vi "SistemaCalentadorAgua.vi"() -> ()   [LabVIEW 2010]
uses:
  <vilib>/Platform/TimedLoop/XDataNode/XDataNode.xnode
  <vilib>/Platform/TimedLoop/XDataNode/timing_clust.ctl
  <vilib>/Platform/TimedLoop/XDataNode/nitl_modes.ctl
  <vilib>/Platform/TimedLoop/XDataNode/wakeup.ctl
  <vilib>/Instr/_visa.llb/VISA Configure Serial Port (Instr).vi
  <vilib>/Platform/TimedLoop/XDataNode/XDNodeRunTimeDep.lvlib
panel:
  out "Waveform Chart 2":i16(graph)
  in  "Ajuste":i16(slide) scale=0.0..10.0
  out "Waveform Chart":dynamicdata(graph)
  out "Temp Actual":i16(slide) scale=20.0..60.0
  in  "Set- Point\n       Temperatura 2":i16(slide) scale=20.0..60.0
  out "off":bool
  out "on":bool
  in  "Manual/Automatico":bool
  in  "Set- Point Potencia (W)":i16(slide) scale=0.0..400.0
  out "valvula":bool
  out "Caldera":dbl(slide) scale=0.0..10.0
  in  "Period                :":i64=1000
  in  "Flow control    :":u16(ring) items=["None"=0, "XON/XOFF"=1, "RTS/CTS"=2, "DTR/DSR"=4]
  in  "Stop bits         :":u16(ring)=10 items=["1.0"=10, "1.5"=15, "2.0"=20]
  in  "Paridad            :":u16(ring) items=["None", "Odd", "Even", "Mark", "Space"]
  in  "Data bits          :":u16=8 min=5 max=8 step=1
  in  "VISA resource : name:":refnum<visa-resource-name>="COM1"
  in  "Baud rate         :":u32=9600
  in  "stop":bool
  out "Read buffer":string
  out "var t":i32
  # "Calentador de Agua"
  # "Configuracion Serial"
  # "Valvula"
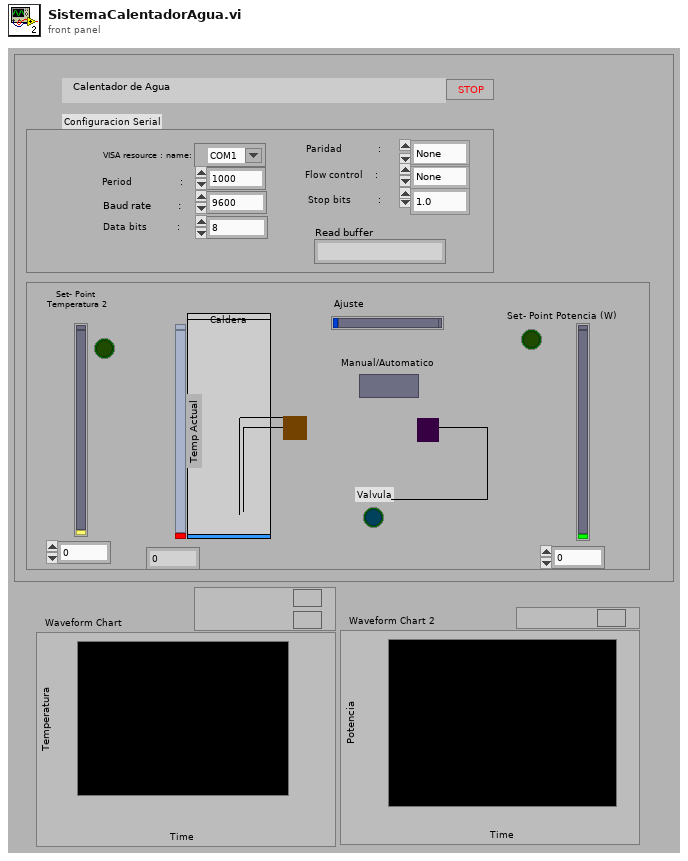
[diagram p1: front panel]
types:
  T1 = typedef "XDNodeRunTimeDep.lvlib/timing_clust.ctl" = cluster{"Expected End [f-1]":u64, "Actual End [f-1]":u64, "Finished Late? [f-1]":bool, "Expected End [i-1]":u64, "Actual End [i-1]":u64, "Finished Late? [i-1]":bool, "Expected Start [i]":u64, "Actual Start [i]":u64, "Expected Start [f]":u64, "Actual Start [f]":u64, "Source Name":string, "Structure Name":string, "Period":i64, "Deadline":i64, "Offset":i64, "Start":i64, "Priority":i32, "Timeout":i32, "Mode":T2, "Wakeup Reason":T3, "Error":errorcluster, "Source Type":string, "Secondary Source Type":string, "Global End Time":u64, "Global Start Time":u64, "Frame Duration":u64, "Iteration Duration":u64, "Assigned CPU":i32, "I/O Scan Engine Mode":u32}
  T2 = typedef "XDNodeRunTimeDep.lvlib/nitl_modes.ctl" = enum32{"No Change", "Process missed periods, maintain original phase", "Discard missed periods, maintain original phase", "Process missed periods, ignore original phase", "Discard missed periods, ignore original phase"}
  T3 = typedef "XDNodeRunTimeDep.lvlib/wakeup.ctl" = enum32{"Normal", "Aborted", "Asynchronous wakeup", "Timing source error", "Timed loop error", "Timeout"}
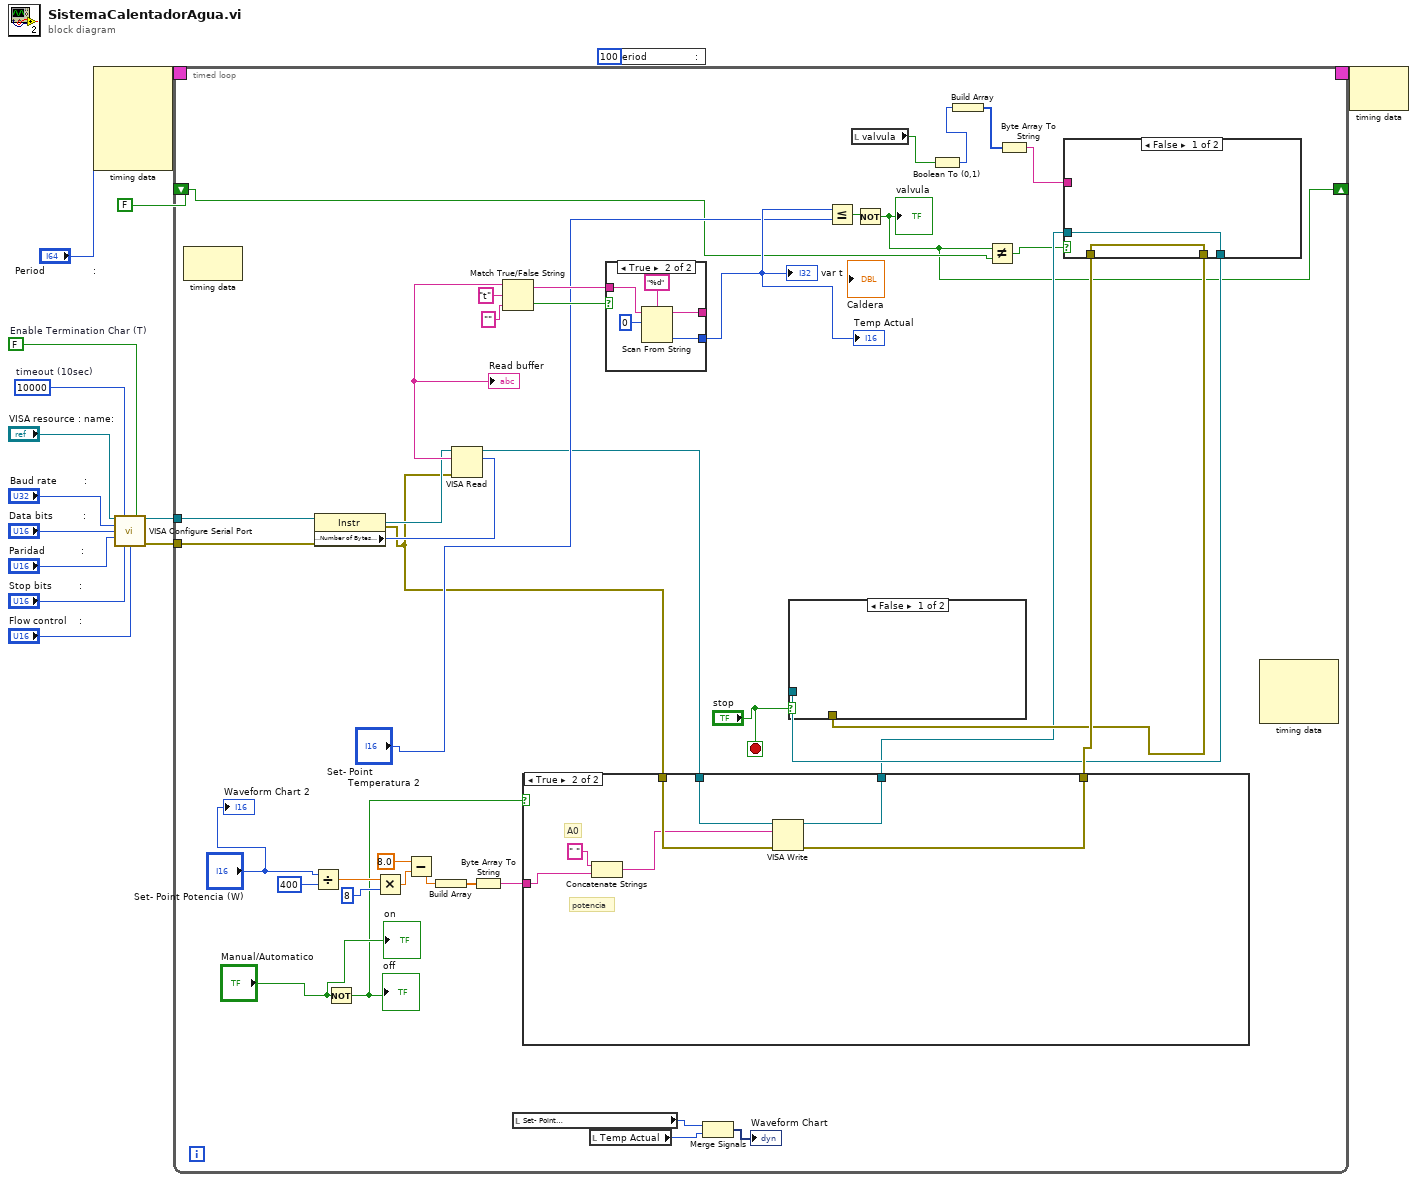
[diagram p0: block diagram]
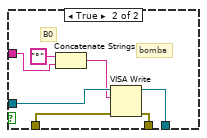
[diagram p2: hidden frame]
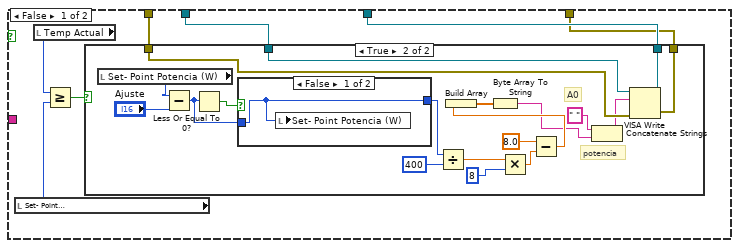
[diagram p3: hidden frame]
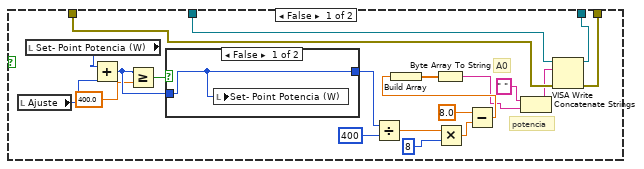
[diagram p4: hidden frame]
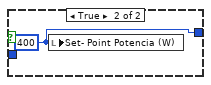
[diagram p5: hidden frame]
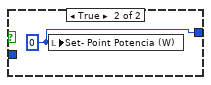
[diagram p6: hidden frame]
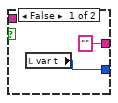
[diagram p7: hidden frame]
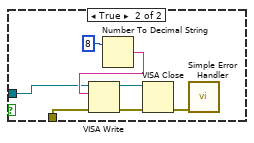
[diagram p8: hidden frame]
diagram:
  w9 = FALSE  # Enable Termination Char (T)
  w10 = u32 10000  # timeout (10sec)
  n1 = node-c288("Period                :") -> (w15:T1)  [unwired: 4 in]
  n2 = call-poly "VISA Configure Serial Port"("VISA resource name"="VISA resource : name:", "timeout (10sec)"=w10, "Enable Termination\nChar (T)"=w9, "baud rate (9600)"="Baud rate         :", "data bits (8)"="Data bits          :", "parity (0:none)"="Paridad            :", "stop bits (10: 1 bit)"="Stop bits         :", "flow control (0:none)"="Flow control    :") -> ("VISA resource name out"=w5:refnum<visa-resource-name>, "error out"=w4:errorcluster)  [unwired: 6 in]
  n3 = timed-loop {
    timing: w15 -> [_]
    timing-out: [_] -> w14
    tunnel: w5 -> [w47]
    tunnel: w4 -> [w46]
    shift-right: [w17] -> _
    shift-left: FALSE -> [w18]
    stop <- "stop" stop-if-true
    n4 = node-c288() -> ()  [unwired: 1 in, 1 out]
    n5 = Divide(x="Set- Point Potencia (W)", y=u16 400) -> (x/y=w43:dbl)
    n6 = property class="Instr"(reference=w47, error in=w46) -> (reference out=w48:refnum<visa-resource-name>, error out=w25:errorcluster, "Serial Settings:Number of Bytes at Serial Port"=w55:u32)
    n7 = Not(x="Manual/Automatico") -> (.not. x?=w36:bool)
    "off" <- w36
    n8 = Multiply(x=w43, y=8) -> (x*y=w35:dbl)
    n9 = Subtract(x=8.0, y=w35) -> (x-y=w33:dbl)
    n10 = Build Array(w33) -> (w41:dbl[])
    n11 = VISA Read(VISA resource name=w48, byte count=w55, error in (no error)=w25) -> (VISA resource name out=w21:refnum<visa-resource-name>, read buffer=w53:string)  [unwired: 2 out]
    "Read buffer" <- w53
    n12 = Byte Array To String(unsigned byte array=w41) -> (string=w45:string)
    n13 = Match True/False String(2:"" ("false string"), 3:"t" ("true string"), 4:w53) -> (0:w51:bool, 1:w50:string)
    n14 = local read "Set- Point\n       Temperatura 2"() -> (w32:i16)
    n15 = case shown="True" w36 {
      tunnel: w21 -> [w68 w121]
      tunnel: w25 -> [w67 w120]
      tunnel: [w66 w119] -> w20
      tunnel: [w65 w118] -> w24
      tunnel: w45 -> [_ w116]
      frame False {
        n16 = local read "Set- Point\n       Temperatura 2"() -> (w70:i16)
        n17 = local read "Temp Actual"() -> (w71:i16)
        n18 = Greater Or Equal?(x=w71, y=w70) -> (x >= y?=w69:bool)
        n19 = case shown="True" w69 {
          tunnel: w68 -> [w88 w107]
          tunnel: w67 -> [w89 w104]
          tunnel: [w84 w106] -> w66
          tunnel: [w83 w105] -> w65
          frame False {
            # "potencia"
            # "A0"
            n20 = local read "Ajuste"() -> (w75:i16)
            n21 = local read "Set- Point Potencia (W)"() -> (w91:i16)
            n22 = Add(x=w91, y=w75) -> (x+y=w86:i16)
            n23 = Greater Or Equal?(x=w86, y=400.0) -> (x >= y?=w87:bool)
            n24 = case shown="False" w87 {
              tunnel: [w92 w93] -> w77
              tunnel: w86 -> [w92 _]
              frame False {
                n25 = local write "Set- Point Potencia (W)"(w92) -> ()
              }
              frame True {
                w93 = u16 400 ("Set- Point Potencia (W)")
                n26 = local write "Set- Point Potencia (W)"(w93) -> ()
              }
            }
            n27 = Divide(x=w77, y=u16 400) -> (x/y=w81:dbl)
            n28 = Multiply(x=w81, y=8) -> (x*y=w79:dbl)
            n29 = Subtract(x=8.0, y=w79) -> (x-y=w76:dbl)
            n30 = Build Array(w76) -> (w90:dbl[])
            n31 = Byte Array To String(unsigned byte array=w90) -> (string=w73:string)
            n32 = Concatenate Strings(" " ("string"), w73) -> (w72:string)
            n33 = VISA Write(VISA resource name=w88, write buffer=w72, error in (no error)=w89) -> (VISA resource name out=w84:refnum<visa-resource-name>, error out=w83:errorcluster)  [unwired: 1 out]
          }
          frame True {
            # "potencia"
            # "A0"
            n34 = local read "Set- Point Potencia (W)"() -> (w112:i16)
            n35 = Subtract(x=w112, y="Ajuste") -> (x-y=w108:i16)
            n36 = Less Or Equal To 0?(x=w108) -> (x <= 0?=w110:bool)
            n37 = case shown="False" w110 {
              tunnel: [w113 w114] -> w98
              tunnel: w108 -> [w113 _]
              frame False {
                n38 = local write "Set- Point Potencia (W)"(w113) -> ()
              }
              frame True {
                w114 = u16 0 ("Set- Point Potencia (W)")
                n39 = local write "Set- Point Potencia (W)"(w114) -> ()
              }
            }
            n40 = Divide(x=w98, y=u16 400) -> (x/y=w102:dbl)
            n41 = Multiply(x=w102, y=8) -> (x*y=w100:dbl)
            n42 = Subtract(x=8.0, y=w100) -> (x-y=w97:dbl)
            n43 = Build Array(w97) -> (w109:dbl[])
            n44 = Byte Array To String(unsigned byte array=w109) -> (string=w95:string)
            n45 = Concatenate Strings(" " ("string"), w95) -> (w94:string)
            n46 = VISA Write(VISA resource name=w107, write buffer=w94, error in (no error)=w104) -> (VISA resource name out=w106:refnum<visa-resource-name>, error out=w105:errorcluster)  [unwired: 1 out]
          }
        }
      }
      frame True {
        # "potencia"
        # "A0"
        n47 = Concatenate Strings(" " ("string"), w116) -> (w117:string)
        n48 = VISA Write(VISA resource name=w121, write buffer=w117, error in (no error)=w120) -> (VISA resource name out=w119:refnum<visa-resource-name>, error out=w118:errorcluster)  [unwired: 1 out]
      }
    }
    n49 = local read "Temp Actual"() -> (w31:i16)
    n50 = case shown="True" w51 {
      tunnel: w50 -> [_ w126]
      tunnel: [w123 w125] -> w40
      tunnel: ["" w124] -> _
      frame False {
        n51 = local read "var t"() -> (w123:i32)
      }
      frame True {
        n52 = Scan From String(format string="%d", input string=w126, initial scan location=u32 0) -> (remaining string=w124:string, output 1=w125:i32)  [unwired: 2 in, 2 out]
      }
    }
    "var t" <- w40
    "Temp Actual" <- w40
    n53 = Merge Signals(w32, w31) -> (→"Waveform Chart":dynamicdata)
    n54 = Less Or Equal?(x=w40, y="Set- Point\n       Temperatura 2") -> (x <= y?=w38:bool)
    n55 = local read "valvula"() -> (w16:bool)
    n56 = Not(x=w38) -> (.not. x?=w17:bool)
    "valvula" <- w17
    n57 = Boolean To (0,1)(Boolean=w16) -> (0, 1=w28:i16)
    n58 = Build Array(w28) -> (w27:i16[])
    n59 = Not Equal?(x=w17, y=w18) -> (x != y?=w19:bool)
    n60 = Byte Array To String(unsigned byte array=w27) -> (string=w26:string)
    n61 = case shown="False" w19 {
      tunnel: w26 -> [_ w61]
      tunnel: w24 -> [w56 w64]
      tunnel: w20 -> [w57 w63]
      tunnel: [w56 w59] -> w23
      tunnel: [w57 w58] -> w22
      frame False {
      }
      frame True {
        # "bomba"
        # "B0"
        n62 = Concatenate Strings("°" ("string"), w61) -> (w60:string)
        n63 = VISA Write(VISA resource name=w63, write buffer=w60, error in (no error)=w64) -> (VISA resource name out=w58:refnum<visa-resource-name>, error out=w59:errorcluster)  [unwired: 1 out]
      }
    }
    n64 = case shown="False" "stop" {
      tunnel: w22 -> [_ w130]
      tunnel: w23 -> [_ w129]
      frame False {
      }
      frame True {
        n65 = Number To Decimal String(number=8) -> (decimal integer string=w131:string)  [unwired: 1 in]
        n66 = VISA Write(VISA resource name=w130, write buffer=w131, error in (no error)=w129) -> (VISA resource name out=w133:refnum<visa-resource-name>, error out=w132:errorcluster)  [unwired: 1 out]
        n67 = VISA Close(VISA resource name=w133, error in (no error)=w132) -> (error out=w135:errorcluster)
        n68 = call <vilib>:"Simple Error Handler.vi"("error in (no error)"=w135) -> ()  [unwired: 4 in, 5 out]
      }
    }
    n69 = node-c288() -> ()  [unwired: 3 in, 1 out]
    "on" <- "Manual/Automatico"
    "Waveform Chart 2" <- "Set- Point Potencia (W)"
  }
  n70 = local write "Period                :"(i64 100 ("Period")) -> ()
  n71 = node-c288(w14) -> ()  [unwired: 1 out]
